vi "ReAddNoise.vi"(1 "Data in":i16[][](array[numeric])=[[1, 2, 2, 3, 4], [2, 3, 3, 0, 0], [1, 1, 2, 3, 4]]) -> (0 "Data out":i16[][](array[numeric]))   [LabVIEW 2022 SP3]
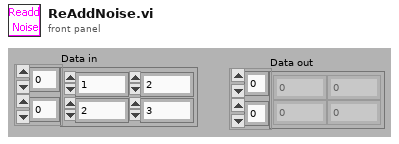
[diagram p1: front panel]
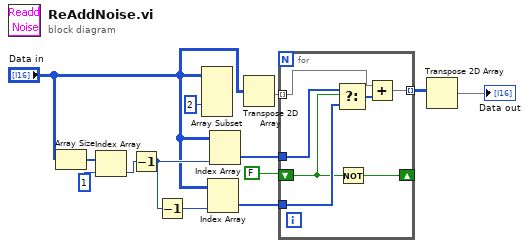
[diagram p0: block diagram]
diagram:
  n1 = Array Size(array="Data in") -> (size(s)=w10:i32[])
  n2 = Index Array(array=w10, index=1) -> (element=w9:i32)
  n3 = Decrement(x=w9) -> (x-1=w8:i32)
  n4 = Decrement(x=w8) -> (x-1=w7:i32)
  n5 = Array Subset(array="Data in", index (col)=2) -> ()  [unwired: 3 in, 1 out]
  n6 = Index Array(array="Data in", index (col)=w7) -> (element=w2:i16[])  [unwired: 1 in]
  n7 = Index Array(array="Data in", index (col)=w8) -> (element=w3:i16[])  [unwired: 1 in]
  n8 = Transpose 2D Array(2D array="Data in") -> (transposed array=w13:i16[][])
  n9 = for {
    tunnel: w13 -> [w17] mode=indexing
    tunnel: w3 -> [w20]
    tunnel: w2 -> [w19]
    tunnel: [w16] -> w5 mode=indexing
    shift-right: [w14] -> _
    shift-left: FALSE -> [w15]
    n10 = Select(t=w20, s=w15, f=w19) -> (s? t:f=w18:i16[])
    n11 = Not(x=w15) -> (.not. x?=w14:bool)
    n12 = Add(x=w17, y=w18) -> (x+y=w16:i16[])
  }
  n13 = Transpose 2D Array(2D array=w5) -> (transposed array=→"Data out":i16[][])
